vi "Signal_Out_Switch(S3).vi"(8 "error in":errorcluster, 10 "Output":T1(ring)=enum."2 Watt Term (TM3)", 11 "Input":T2(ring)=enum."IO Switch #1 (S1)") -> (0 "error out":errorcluster, 2 "Verfied":bool, 3 "Switches":string)   [LabVIEW 2012]
panel:
  # "Signal Out Switch (S3)"
  # "Switch Output"
  # "Switch Input"
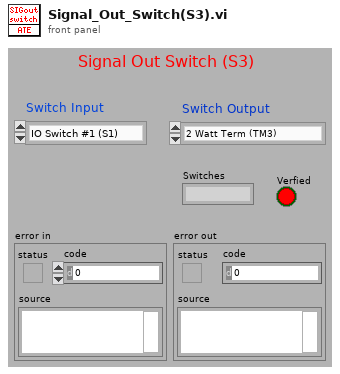
[diagram p1: front panel]
types:
  T1 = enum16{"NONE", "2 Watt Term (TM3)", "Splitter", "Power Meter Switch (S5)"}
  T2 = enum16{"NONE", "Amp Bypass Switch (S6)", "IO Switch #1 (S1)", "IO Switch #2 (S2)", "2W Term (TM3)"}
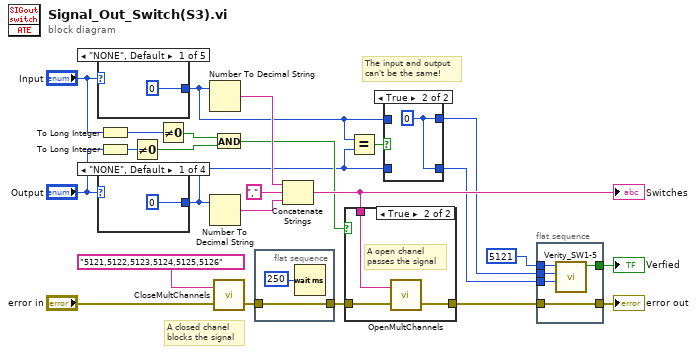
[diagram p0: block diagram]
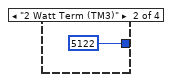
[diagram p3: hidden frame]
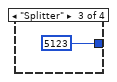
[diagram p4: hidden frame]
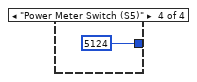
[diagram p5: hidden frame]
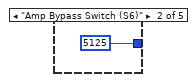
[diagram p6: hidden frame]
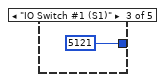
[diagram p7: hidden frame]
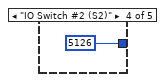
[diagram p8: hidden frame]
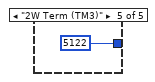
[diagram p9: hidden frame]
diagram:
  # "The input and output\ncan't be the same!"
  # "A closed chanel\nblocks the signal"
  n1 = case shown="\"NONE\", Default" "Input" {
    tunnel: [0 ("Switch ID") 5125 ("Switch ID") 5121 ("Switch ID") 5126 ("Switch ID") 5122 ("Switch ID")] -> w6
    frame "NONE", Default {
    }
    frame "Amp Bypass Switch (S6)" {
    }
    frame "IO Switch #1 (S1)" {
    }
    frame "IO Switch #2 (S2)" {
    }
    frame "2W Term (TM3)" {
    }
  }
  n2 = case shown="\"NONE\", Default" "Output" {
    tunnel: [0 ("Switch ID") 5122 ("Switch ID") 5123 ("Switch ID") 5124 ("Switch ID")] -> w5
    frame "NONE", Default {
    }
    frame "2 Watt Term (TM3)" {
    }
    frame "Splitter" {
    }
    frame "Power Meter Switch (S5)" {
    }
  }
  n3 = To Long Integer(number="Input") -> (32bit integer=w14:i32)
  n4 = To Long Integer(number="Output") -> (32bit integer=w13:i32)
  n5 = Not Equal To 0?(x=w13) -> (x != 0?=w12:bool)
  n6 = Not Equal To 0?(x=w14) -> (x != 0?=w11:bool)
  n7 = Number To Decimal String(number=w6) -> (decimal integer string=w17:string)  [unwired: 1 in]
  n8 = Number To Decimal String(number=w5) -> (decimal integer string=w18:string)  [unwired: 1 in]
  n9 = And(x=w11, y=w12) -> (x .and. y?=w10:bool)
  n10 = call "CloseMultChannels.vi"("error in (no error)"="error in", "Channels to be closed"="5121,5122,5123,5124,5125,5126" ("Channels to be opened")) -> ("error out"=w20:errorcluster)  [unwired: 1 in]
  n11 = flat-sequence {
    tunnel: w20 -> [w34]
    tunnel: [w34] -> w19
    frame #0 {
      n12 = Wait (ms)(milliseconds to wait=u32 250) -> ()  [unwired: 1 out]
    }
  }
  n13 = Concatenate Strings(w17, ",", w18) -> (w21:string)
  "Switches" <- w21
  n14 = case shown="True" w10 {
    tunnel: w19 -> [w36 w38]
    tunnel: w21 -> [_ w39]
    tunnel: [w36 w37] -> w4
    frame False {
    }
    frame True {
      # "A open chanel\npasses the signal"
      n15 = call "OpenMultChannels.vi"("error in (no error)"=w38, "Channels to be opened"=w39) -> ("error out"=w37:errorcluster)  [unwired: 1 in]
    }
  }
  n16 = Equal?(x=w6, y=w5) -> (x = y?=w7:bool)
  n17 = case shown="True" w7 {
    tunnel: w5 -> [w40 _]
    tunnel: [w40 w42] -> w2
    tunnel: w6 -> [w41 _]
    tunnel: [w41 w42] -> w1
    frame False {
    }
    frame True {
      w42 = 0 ("Switch ID")
    }
  }
  n18 = flat-sequence {
    tunnel: 5121 ("Switch ID") -> [w47]
    tunnel: w1 -> [w46]
    tunnel: w2 -> [w45]
    tunnel: [w44] -> w9
    tunnel: w4 -> [w43]
    tunnel: [w43] -> w3
    frame #0 {
      n19 = call "Verity_SW1-5.vi"("Output Switch ID"=w45, "Input Switch ID"=w46, "Base Switch ID"=w47) -> ("Verfied"=w44:bool)  [unwired: 7 in, 1 out]
    }
  }
  "error out" <- w3
  "Verfied" <- w9
